vi "TSPopup.Update Cell String.vi"(8 "error in (no error)":errorcluster, 9 "Call Data (must be Cell Info cluster)":variant, 11 "Popup Value":variant) -> (0 "error out":errorcluster)   [LabVIEW 2016, in "TSPopup.lvlib" / "TSPopup.lvclass"]
doc: "Changes the text of the location that was clicked on to reflect whatever is contained in <B>Popup Value</B>. This subVI must be used in the <Popup Event> event, which provides the needed inputs.\n<B>NOTE</B> : This only works if the Cell Info cluster was used directly as the Call Data.\n\n<B>Popup Value</B> - Value entered into the Type Sensitive Popup.\n<B>Call data</B> - Call data returned by <Popup Event> event (must be the Cell Info cluster).\n\nType Sensitive Popup \nCopyright © 2007, J. David Saunders\nAll rights reserved."
uses:
  <userlib>/TSPopup/TSPopup.lvclass
  <userlib>/TSPopup/TSPopup.Grid.Cell Info.ctl
  <userlib>/TSPopup/TSPopup.Data Type.ctl
panel:
  in  "rect":T1
  in  "point":cluster{"x":i16, "y":i16}
  in  "Cell Info (type only)":T2
  # "Type Sensitive Popup \nCopyright © 2007, J. David Saunders\nAll rights reserved."
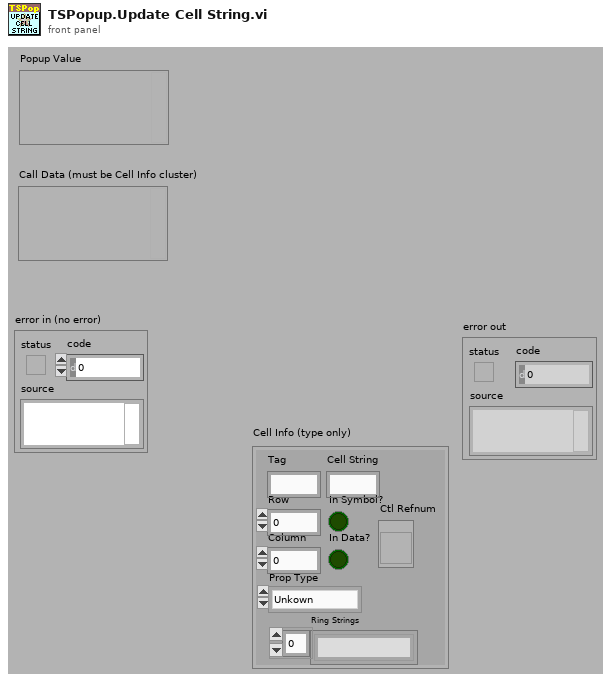
[diagram p1: front panel]
types:
  T1 = cluster{"left":i16, "top":i16, "right":i16, "bottom":i16}
  T2 = typedef "TSPopup.lvlib/TSPopup.lvclass/TSPopup.Grid.Cell Info.ctl" = cluster{"Tag":string, "Row":i32, "Column":i32, "In Symbol?":bool, "In Data?":bool, "Cell String":string, "Ctl Refnum":refnum<vi>, "Prop Type":T3, "Ring Strings":string[]}
  T3 = typedef "TSPopup.lvlib/TSPopup.lvclass/TSPopup.Data Type.ctl" = enum16{"Unkown", "NO POPUP", "String", "Integer", "Float", "Color", "Boolean", "Ring", "Captioned String", "Captioned Integer", "Button Color", "2 Int Cluster", "4 Int Cluster", "check"}
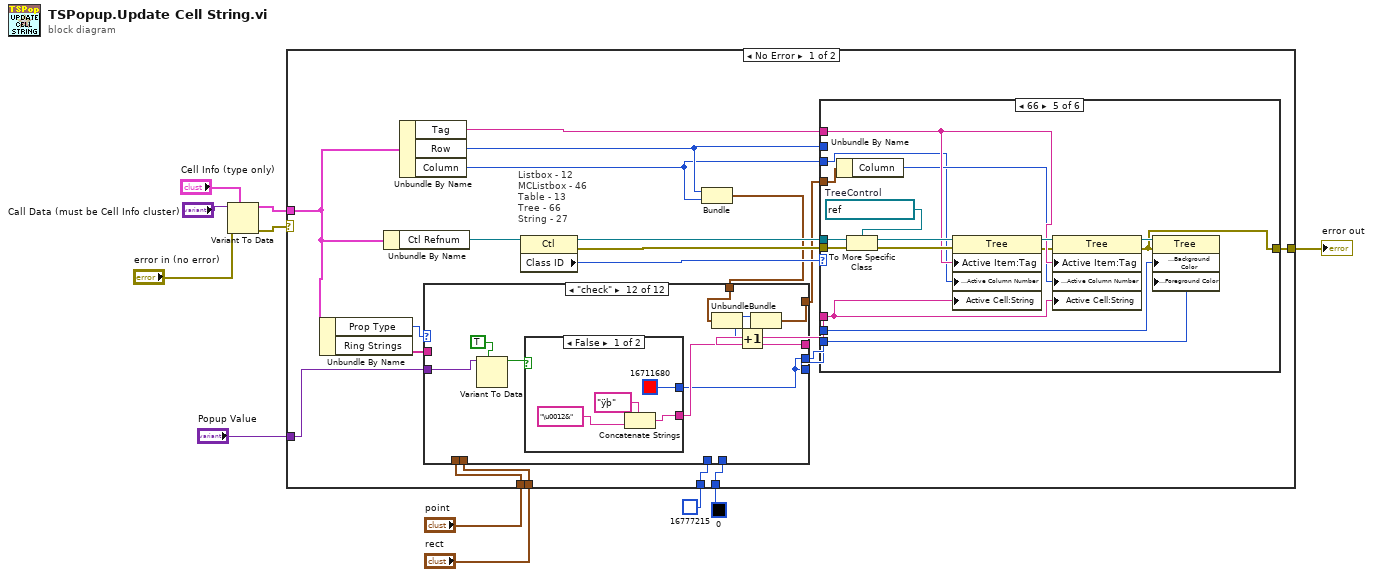
[diagram p0: block diagram]
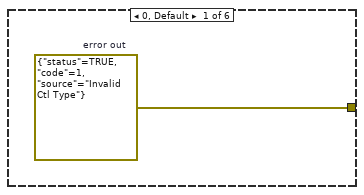
[diagram p2: hidden frame]
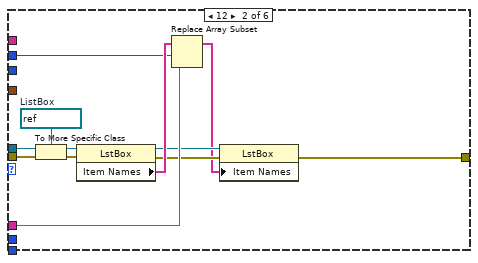
[diagram p3: hidden frame]
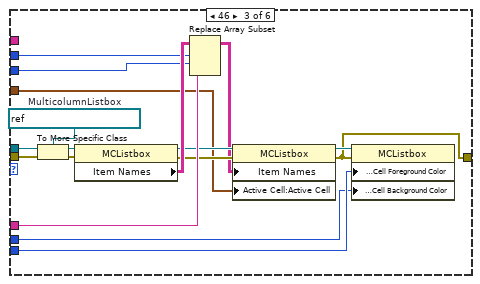
[diagram p4: hidden frame]
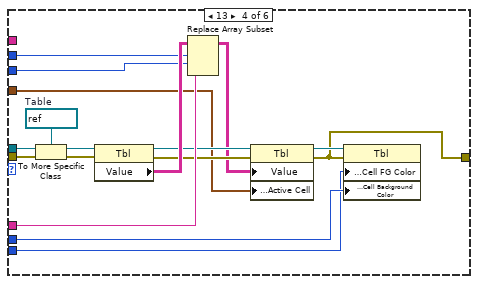
[diagram p5: hidden frame]
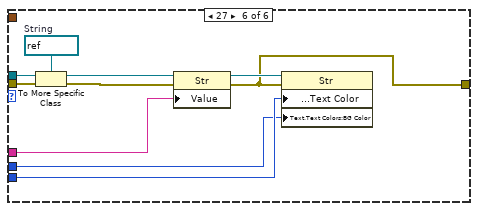
[diagram p6: hidden frame]
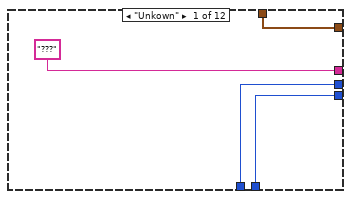
[diagram p7: hidden frame]
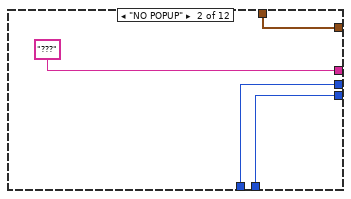
[diagram p8: hidden frame]
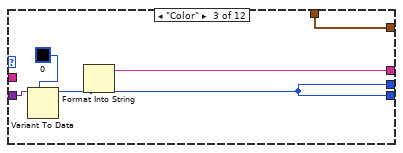
[diagram p9: hidden frame]
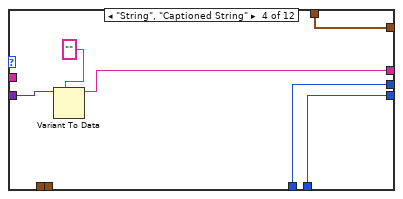
[diagram p10: hidden frame]
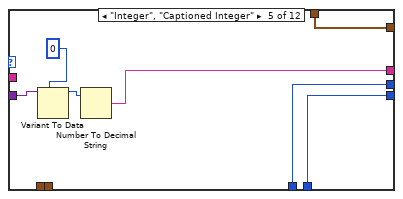
[diagram p11: hidden frame]
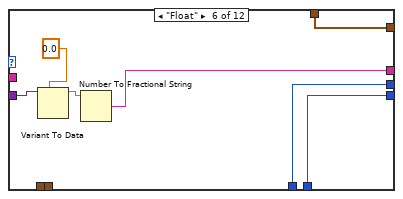
[diagram p12: hidden frame]
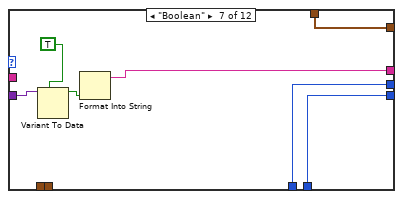
[diagram p13: hidden frame]
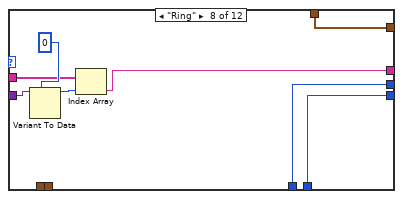
[diagram p14: hidden frame]
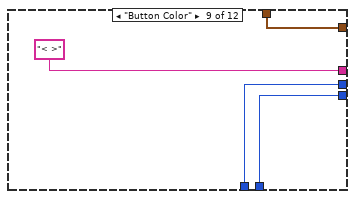
[diagram p15: hidden frame]
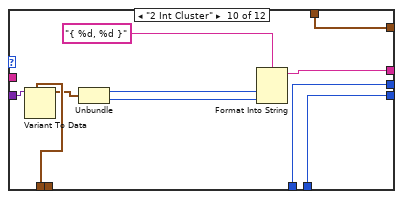
[diagram p16: hidden frame]
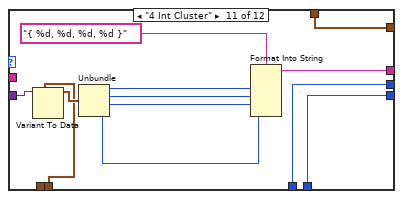
[diagram p17: hidden frame]
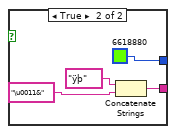
[diagram p18: hidden frame]
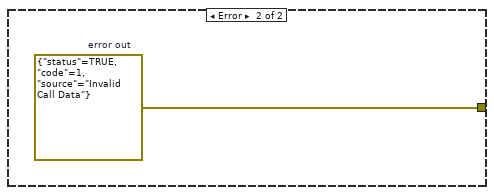
[diagram p19: hidden frame]
diagram:
  n1 = Variant To Data(error in="error in (no error)", type="Cell Info (type only)", Variant="Call Data (must be Cell Info cluster)") -> (data=w9:T2, error out=w7:errorcluster)
  n2 = case shown="No Error" w7 {
    tunnel: w9 -> [w26 _]
    tunnel: [w27 w198] -> w8
    tunnel: "Popup Value" -> [w21 _]
    tunnel: "point" -> [w15 _]
    tunnel: "rect" -> [w14 _]
    tunnel: u32 0 -> [w17 _]
    tunnel: u32 16777215 -> [w16 _]
    frame No Error {
      # "Listbox - 12\nMCListbox - 46\nTable - 13\nTree - 66\nString - 27"
      n3 = Unbundle By Name(w26) -> ("Prop Type"=w23:T3, "Ring Strings"=w22:string[])
      n4 = Unbundle By Name(w26) -> ("Ctl Refnum"=w29:refnum<vi>)
      n5 = Unbundle By Name(w26) -> ("Tag"=w28:string, "Row"=w25:i32, "Column"=w24:i32)
      n6 = property class="Ctl"(reference=w29) -> (reference out=w31:refnum<vi>, error out=w30:errorcluster, "Class ID"=w32:u32)  [unwired: 1 in]
      n7 = Bundle("Row"=w25, "Column"=w24) -> (w13:cluster{"Row":i32, "Column":i32})  [unwired: 1 in]
      n8 = case shown="\"check\"" w23 {
        tunnel: w22 -> [_ _ _ _ _ _ _ w151 _ _ _ _]
        tunnel: w21 -> [_ _ w118 w121 w129 w136 w143 w153 _ w167 w179 w188]
        tunnel: ["???" "???" w116 w120 w126 w133 w140 w149 "< >" w161 w175 w186] -> w20
        tunnel: w15 -> [_ _ _ _ _ _ _ _ _ w166 _ _]
        tunnel: w14 -> [_ _ _ _ _ _ _ _ _ _ w174 _]
        tunnel: [w107 w111 w115 w124 w131 w138 w145 w147 w155 w160 w170 w180] -> w18
        tunnel: [w108 w112 w115 w123 w130 w137 w144 w148 w156 w159 w169 w180] -> w19
        tunnel: w17 -> [w107 w111 _ w124 w131 w138 w145 w147 w155 w160 w170 _]
        tunnel: w16 -> [w108 w112 _ w123 w130 w137 w144 w148 w156 w159 w169 _]
        tunnel: w13 -> [w106 w110 w114 w119 w125 w132 w139 w146 w154 w158 w168 w185]
        tunnel: [w106 w110 w114 w119 w125 w132 w139 w146 w154 w158 w168 w183] -> w12
        frame "Unkown" {
        }
        frame "NO POPUP" {
        }
        frame "Color" {
          n9 = Variant To Data(type=u32 0, Variant=w118) -> (data=w115:u32)  [unwired: 1 in, 1 out]
          n10 = Format Into String(w115) -> (resulting string=w116:string)  [unwired: 3 in, 1 out]
        }
        frame "String", "Captioned String" {
          n11 = Variant To Data(type="", Variant=w121) -> (data=w120:string)  [unwired: 1 in, 1 out]
        }
        frame "Integer", "Captioned Integer" {
          n12 = Variant To Data(type=0, Variant=w129) -> (data=w127:i32)  [unwired: 1 in, 1 out]
          n13 = Number To Decimal String(number=w127) -> (decimal integer string=w126:string)  [unwired: 1 in]
        }
        frame "Float" {
          n14 = Variant To Data(type=0.0, Variant=w136) -> (data=w134:dbl)  [unwired: 1 in, 1 out]
          n15 = Number To Fractional String(number=w134) -> (F-format string=w133:string)  [unwired: 3 in]
        }
        frame "Boolean" {
          n16 = Variant To Data(type=TRUE, Variant=w143) -> (data=w141:bool)  [unwired: 1 in, 1 out]
          n17 = Format Into String(w141) -> (resulting string=w140:string)  [unwired: 3 in, 1 out]
        }
        frame "Ring" {
          n18 = Variant To Data(type=0, Variant=w153) -> (data=w150:i32)  [unwired: 1 in, 1 out]
          n19 = Index Array(array=w151, index=w150) -> (element=w149:string)
        }
        frame "Button Color" {
        }
        frame "2 Int Cluster" {
          n20 = Variant To Data(type=w166, Variant=w167) -> (data=w162:cluster{"x":i16, "y":i16})  [unwired: 1 in, 1 out]
          n21 = Unbundle(w162) -> ("x"=w164:i16, "y"=w163:i16)
          n22 = Format Into String(format string="{ %d, %d }" ("String"), w164, w163) -> (resulting string=w161:string)  [unwired: 2 in, 1 out]
        }
        frame "4 Int Cluster" {
          n23 = Variant To Data(type=w174, Variant=w179) -> (data=w176:T1)  [unwired: 1 in, 1 out]
          n24 = Unbundle(w176) -> ("left"=w178:i16, "top"=w177:i16, "right"=w173:i16, "bottom"=w172:i16)
          n25 = Format Into String(format string="{ %d, %d, %d, %d }" ("String"), w178, w177, w173, w172) -> (resulting string=w175:string)  [unwired: 2 in, 1 out]
        }
        frame "check" {
          n26 = Variant To Data(type=TRUE, Variant=w188) -> (data=w187:bool)  [unwired: 1 in, 1 out]
          n27 = case shown="False" w187 {
            tunnel: [w191 w195] -> w186
            tunnel: [u32 16711680 u32 6618880] -> w180
            frame False {
              n28 = Concatenate Strings("ÿþ" ("string"), "\u0012&" ("string")) -> (w191:string)
            }
            frame True {
              n29 = Concatenate Strings("ÿþ" ("string"), "\u0011&" ("string")) -> (w195:string)
            }
          }
          n30 = Unbundle(w185) -> ("Row"=w184:i32, "Column"=w182:i32)
          n31 = Increment(x=w182) -> (x+1=w181:i32)
          n32 = Bundle("Row"=w184, w181) -> (w183:cluster{"Row":i32, i32})  [unwired: 1 in]
        }
      }
      n33 = case shown="66" w32 {
        tunnel: w31 -> [_ w44 w61 w78 w94 w104]
        tunnel: w30 -> [_ w43 w60 w77 w93 w103]
        tunnel: w20 -> [_ w39 w56 w73 w82 w100]
        tunnel: w25 -> [_ w35 w52 w69 _ _]
        tunnel: w24 -> [_ _ w51 w68 w83 _]
        tunnel: w28 -> [_ _ _ _ w85 _]
        tunnel: [w33 w34 w46 w63 w80 w96] -> w27
        tunnel: w18 -> [_ _ w48 w64 w90 w98]
        tunnel: w19 -> [_ _ w47 w65 w89 w97]
        tunnel: w12 -> [_ _ w50 w67 w88 _]
        frame 0, Default {
          w33 = errorcluster {"status"=TRUE, "code"=1, "source"="Invalid Ctl Type"}  # error out
        }
        frame 12 {
          w45 = refnum<vi> refnum  # ListBox
          n34 = To More Specific Class(target class=w45, reference=w44, error in=w43) -> (specific class reference=w42:refnum<vi>, error out=w41:errorcluster)
          n35 = property class="LstBox"(reference=w42, error in=w41) -> (reference out=w38:refnum<vi>, error out=w37:errorcluster, "Item Names"=w40:string[])
          n36 = Replace Array Subset(array=w40, new element=w39, index=w35) -> (w36:string[])
          n37 = property class="LstBox"(reference=w38, error in=w37, "Item Names"=w36) -> (error out=w34:errorcluster)  [unwired: 1 out]
        }
        frame 46 {
          w62 = refnum<vi> refnum  # MulticolumnListbox
          n38 = To More Specific Class(target class=w62, reference=w61, error in=w60) -> (specific class reference=w59:refnum<vi>, error out=w58:errorcluster)
          n39 = property class="MCListbox"(reference=w59, error in=w58) -> (reference out=w55:refnum<vi>, error out=w54:errorcluster, "Item Names"=w57:string[][])
          n40 = Replace Array Subset(array=w57, new element=w56, index (row)=w52, index (col)=w51) -> (w53:string[][])
          n41 = property class="MCListbox"(reference=w55, error in=w54, "Item Names"=w53, "Active Cell:Active Cell"=w50) -> (reference out=w49:refnum<vi>, error out=w46:errorcluster)
          n42 = property class="MCListbox"(reference=w49, error in=w46, "Active Cell:Cell Foreground Color"=w48, "Active Cell:Cell Background Color"=w47) -> ()  [unwired: 2 out]
        }
        frame 13 {
          w79 = refnum<vi> refnum  # Table
          n43 = To More Specific Class(target class=w79, reference=w78, error in=w77) -> (specific class reference=w76:refnum<vi>, error out=w75:errorcluster)
          n44 = property class="Tbl"(reference=w76, error in=w75) -> (reference out=w72:refnum<vi>, error out=w71:errorcluster, "Value"=w74:string[][])
          n45 = Replace Array Subset(array=w74, new element=w73, index (row)=w69, index (col)=w68) -> (w70:string[][])
          n46 = property class="Tbl"(reference=w72, error in=w71, "Value"=w70, "Active Cell:Active Cell"=w67) -> (reference out=w66:refnum<vi>, error out=w63:errorcluster)
          n47 = property class="Tbl"(reference=w66, error in=w63, "Active Cell:Cell FG Color"=w64, "Active Cell:Cell Background Color"=w65) -> ()  [unwired: 2 out]
        }
        frame 66 {
          w95 = refnum<vi> refnum  # TreeControl
          n48 = Unbundle By Name(w88) -> ("Column"=w84:i32)
          n49 = To More Specific Class(target class=w95, reference=w94, error in=w93) -> (specific class reference=w92:refnum<vi>, error out=w91:errorcluster)
          n50 = property class="Tree"(reference=w92, error in=w91, "Active Item:Tag"=w85, "Active Cell:Active Column Number"=w83, "Active Cell:String"=w82) -> (reference out=w87:refnum<vi>, error out=w81:errorcluster)
          n51 = property class="Tree"(reference=w87, error in=w81, "Active Item:Tag"=w85, "Active Cell:Active Column Number"=w84, "Active Cell:String"=w82) -> (reference out=w86:refnum<vi>, error out=w80:errorcluster)
          n52 = property class="Tree"(reference=w86, error in=w80, "Active Cell:Background Color"=w89, "Active Cell:Foreground Color"=w90) -> ()  [unwired: 2 out]
        }
        frame 27 {
          w105 = refnum<vi> refnum  # String
          n53 = To More Specific Class(target class=w105, reference=w104, error in=w103) -> (specific class reference=w102:refnum<vi>, error out=w101:errorcluster)
          n54 = property class="Str"(reference=w102, error in=w101, "Value"=w100) -> (reference out=w99:refnum<vi>, error out=w96:errorcluster)
          n55 = property class="Str"(reference=w99, error in=w96, "Text.Text Colors:Text Color"=w98, "Text.Text Colors:BG Color"=w97) -> ()  [unwired: 2 out]
        }
      }
    }
    frame Error {
      w198 = errorcluster {"status"=TRUE, "code"=1, "source"="Invalid Call Data"}  # error out
    }
  }
  "error out" <- w8
